vi "通信并与其他模块交互 (子VI).vi"() -> ()   [LabVIEW 2016, in "质控单元.lvlib"]
uses:
  <vilib>/Plasmionique/MB Master/MB_Master_TCP/MB_Master_TCP.lvclass
  D:/Program Files (x86)/National Instruments/LabVIEW 2016/vi.lib/Plasmionique/MB Master/MB_Master/MB_Master.lvclass
  <vilib>/Plasmionique/MB Master/MB_Master/MB_Master.lvclass
  <vilib>/Plasmionique/MB Master/MB Master.lvlib
  <vilib>/Utility/config.llb/NI_LVConfig.lvlib
panel:
  out "CODCr测量状态":u16[](array[numeric])
  out "CODMn测量状态":u16[](array[numeric])
  out "总氮测量状态":u16[](array[numeric])
  out "总磷测量状态":u16[](array[numeric])
  out "氨氮测量状态":u16[](array[numeric])
  out "通讯状态":bool
  out "待处理插入数量":i32
  out "元素":cluster{"命令":string}[](array[cluster])
  out "队列中元素数量":i32
  in  "starting address 6":u16
  in  "values 6":u16[](array[numeric])
  in  "starting address 5":u16
  in  "values 5":u16[](array[numeric])
  in  "starting address 4":u16
  in  "values 4":u16[](array[numeric])
  in  "starting address 3":u16
  in  "values 3":u16[](array[numeric])
  in  "starting address 2":u16
  in  "values 2":u16[](array[numeric])
  in  "values":u16[](array[numeric])
  in  "starting address":u16
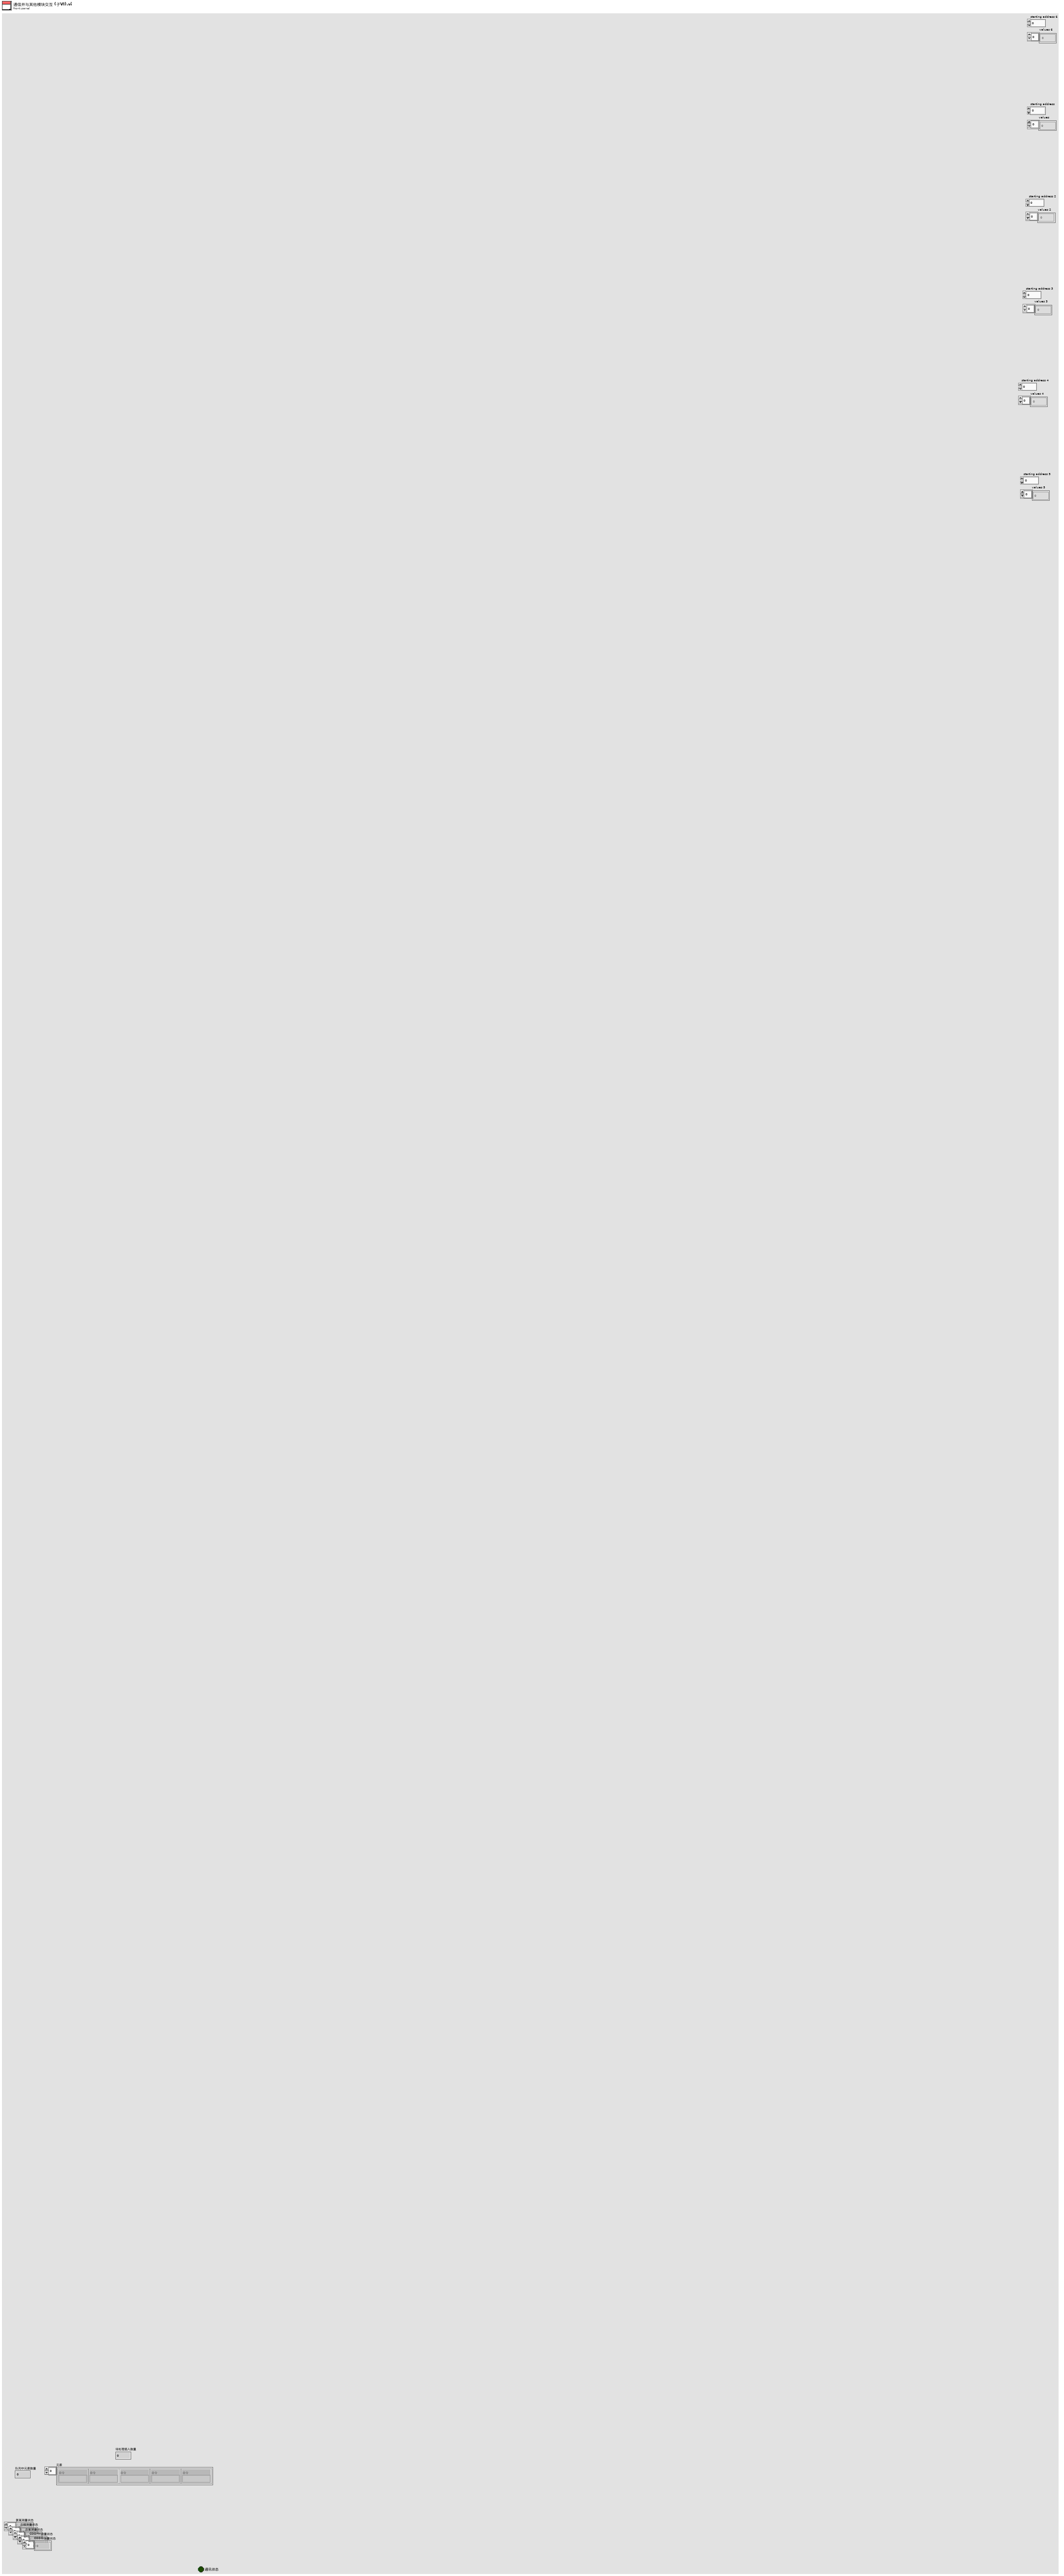
[diagram p1: front panel]
types:
  T1 = typedef "NI_LVConfig.lvlib/Config Data RefNum.ctl" = refnum<k1>
  T2 = cluster{"因子编码":u32, "单位":u16, "标样参考值":sgl, "水样数据时间":timestamp, "水样实测值":sgl, "水样数据标识":string, "标样数据时间":timestamp, "标样实测值":sgl, "标样数据标识":string, "空白数据时间":timestamp, "空白实测值":sgl, "空白数据标识":string, "零点核查数据时间":timestamp, "零点核查实测值":sgl, "零点核查数据标识":string, "跨度核查数据时间":timestamp, "跨度核查实测值":sgl, "跨度核查数据标识":string, "加标回收数据时间":timestamp, "加标回收实测值":sgl, "加标回收数据标识":string, "平行样数据时间":timestamp, "平行样实测值":sgl, "平行样数据标识":string}
  T3 = cluster{"系统时间":timestamp, "工作状态":enum16{"空闲", "水样测试", "标样核查", "零点核查", "跨度核查", "空白测试", "平行样测试", "加标回收", "空白校准", "标样校准", "初始化（清洗）"}, "测量模式":enum16{"待机", "连续模式", "周期模式", "定点模式", "受控模式", "手动模式"}, "告警代码":enum16{"无告警", "缺试剂告警", "缺水样告警", "缺蒸馏水告警", "缺标液告警", "仪表漏液告警", "标定异常告警", "超量程告警", "加热异常", "低试剂预警", "超上限告警", "超下限告警", "仪表内部其他异常", "滴定异常告警", "电极异常告警", "量程切换告警", "参数设置告警", "PH电极电位异常", "电导率电极异常", "浊度光度异常", "溶解氧电极异常", "溶解氧光强异常", "温度异常告警", "PH异常告警", "溶解氧异常告警", "电导率异常告警", "浊度异常告警", "叶绿素异常告警", "藻密度异常告警", "蓝绿藻异常告警", "ORP异常告警", "氨氮异常告警", "清洁刷异常告警", "SD卡异常告警", "蓝牙异常告警", "Wifi异常告警", "流程异常告警"}, "故障代码":enum16{"无故障", "电机故障", "温度故障", "通讯故障", "滴定故障"}, "日志代码":u16, "软件版本":u16, "F0":sgl, "F1":sgl, "F2":sgl, "F3":sgl, "T":sgl, "H":sgl, "id":u16, "flowid":u16, "量程":u16, "总磷控温温度1":sgl, "营养盐控温温度2":sgl, "ADC":sgl}
  T4 = cluster{"Registers[0]":u16, "Registers[1]":u16, "Registers[2]":u16, "Registers[3]":u16, "Registers[4]":u16, "Registers[5]":u16, "Registers[6]":u16, "Registers[7]":u16, "Registers[8]":u16, "Registers[9]":u16, "Registers[10]":u16, "Registers[11]":u16, "Registers[12]":u16, "Registers[13]":u16, "Registers[14]":u16, "Registers[15]":u16, "Registers[16]":u16, "Registers[17]":u16, "Registers[18]":u16, "Registers[19]":u16, "Registers[20]":u16, "Registers[21]":u16, "Registers[22]":u16, "Registers[23]":u16, "Registers[24]":u16, "Registers[25]":u16, "Registers[26]":u16, "Registers[27]":u16, "Registers[28]":u16, "Registers[29]":u16, "Registers[30]":u16, "Registers[31]":u16, "Registers[32]":u16, "Registers[33]":u16, "Registers[34]":u16, "Registers[35]":u16, "Registers[36]":u16, "Registers[37]":u16, "Registers[38]":u16, "Registers[39]":u16, "Registers[40]":u16, "Registers[41]":u16, "Registers[42]":u16, "Registers[43]":u16, "Registers[44]":u16, "Registers[45]":u16, "Registers[46]":u16, "Registers[47]":u16, "Registers[48]":u16, "Registers[49]":u16, "Registers[50]":u16, "Registers[51]":u16, "Registers[52]":u16, "Registers[53]":u16, "Registers[54]":u16, "Registers[55]":u16, "Registers[56]":u16}
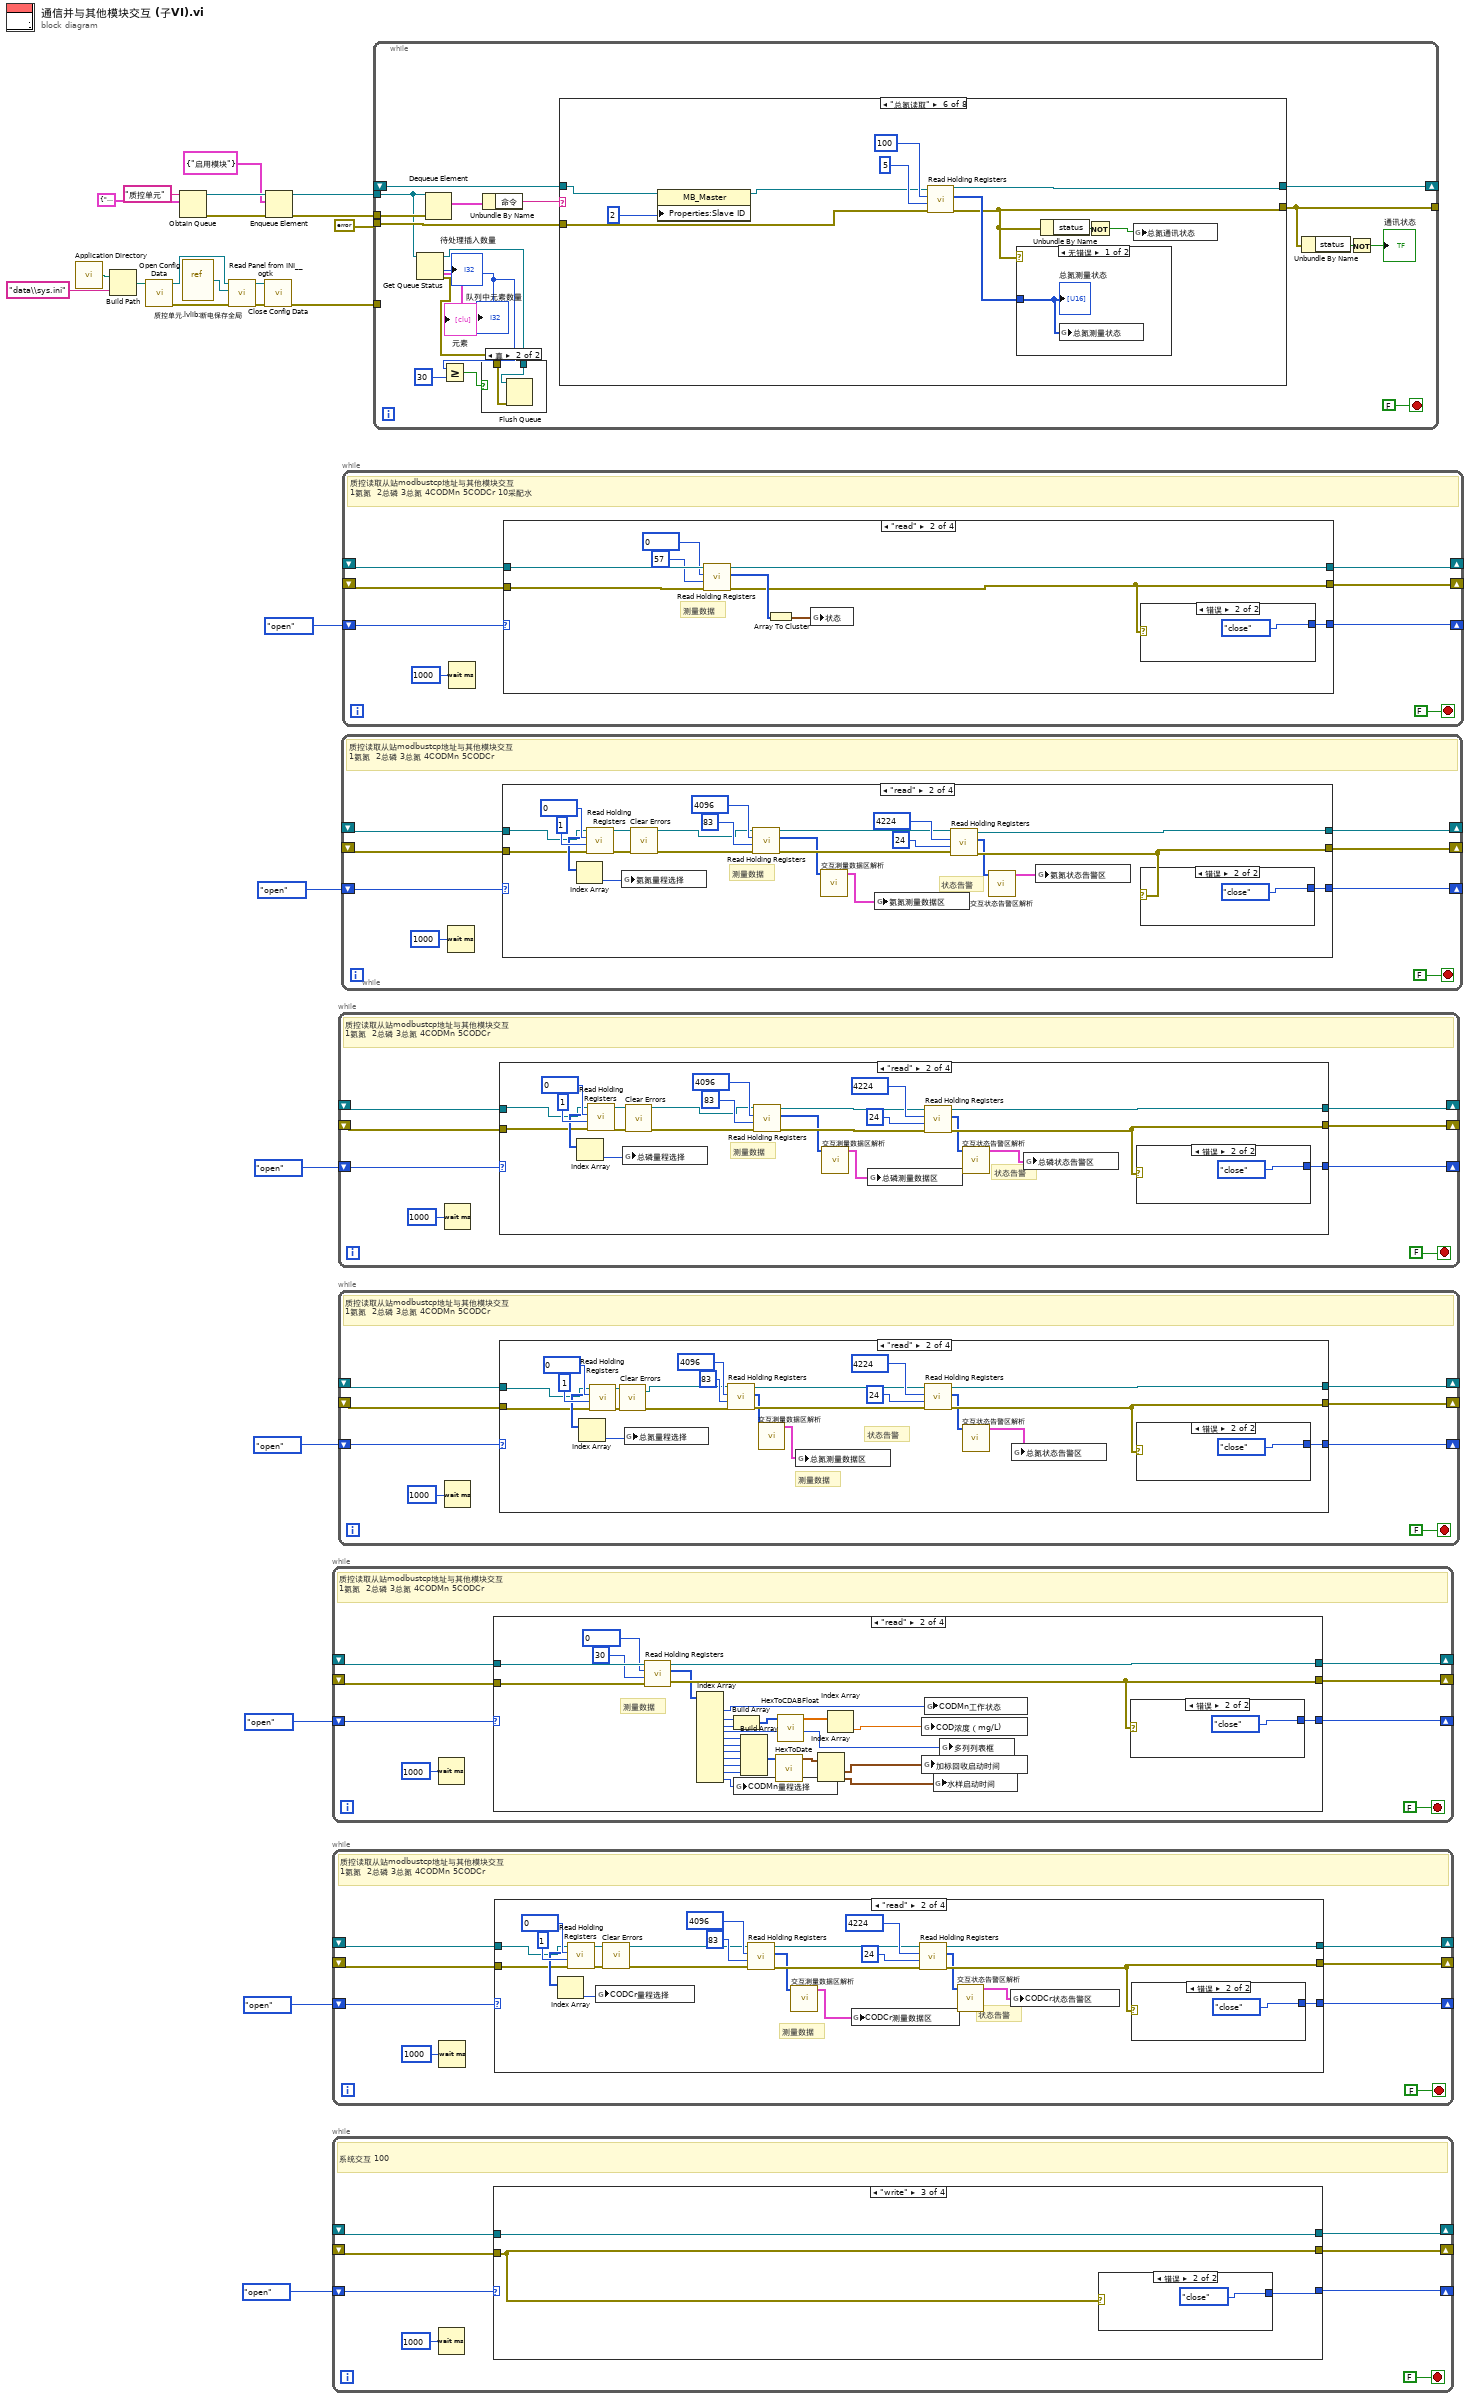
[diagram p0: block diagram]
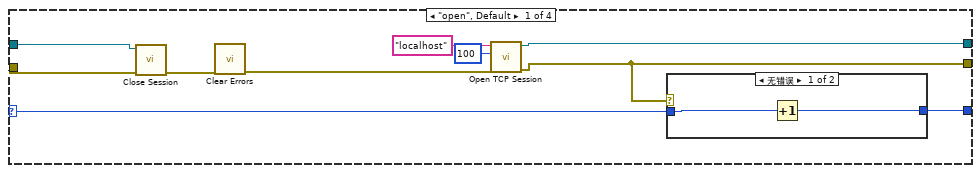
[diagram p2: hidden frame]
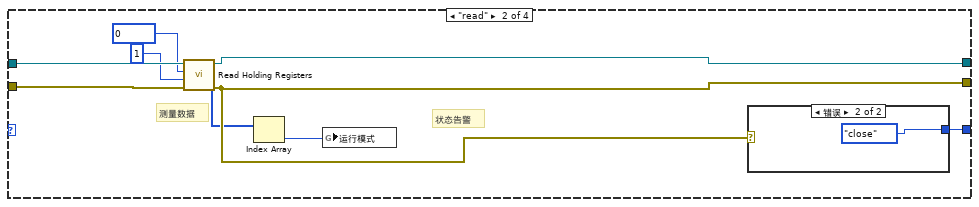
[diagram p4: hidden frame]
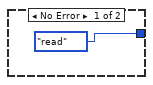
[diagram p5: hidden frame]
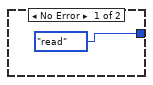
[diagram p6: hidden frame]
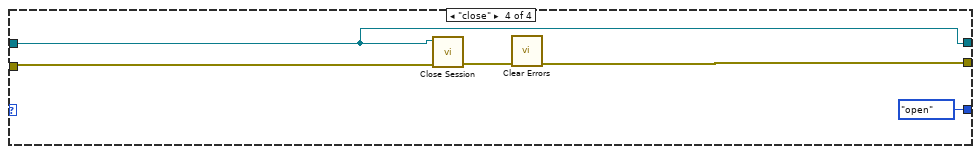
[diagram p7: hidden frame]
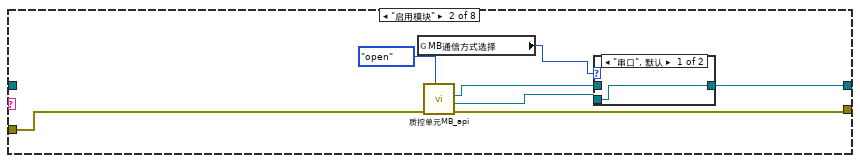
[diagram p10: hidden frame]
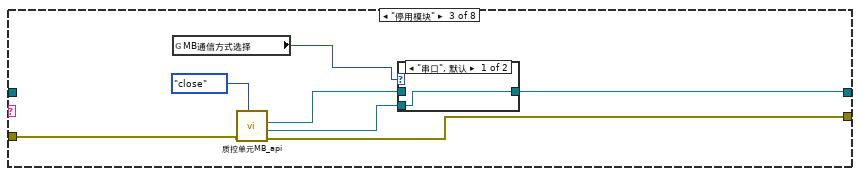
[diagram p12: hidden frame]
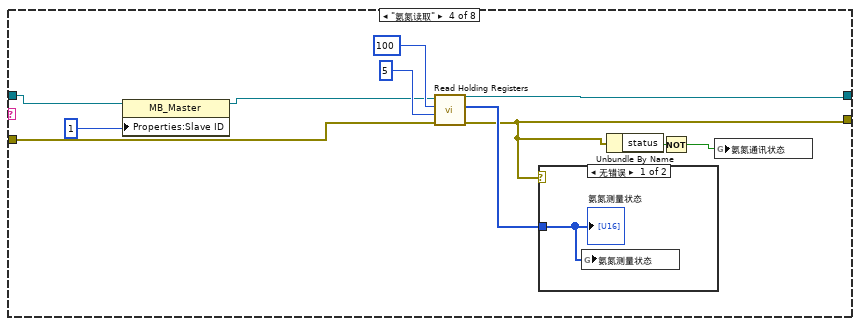
[diagram p14: hidden frame]
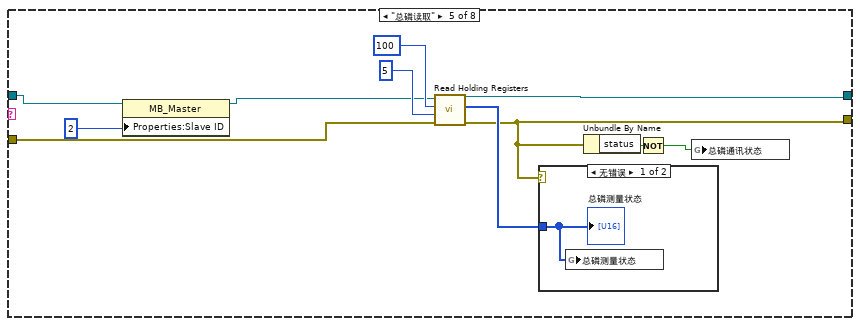
[diagram p16: hidden frame]
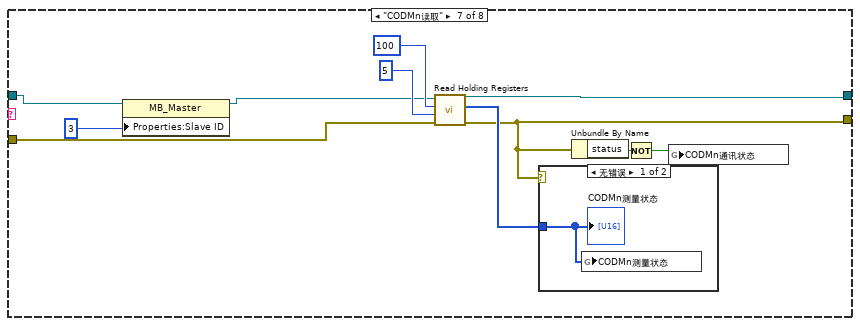
[diagram p19: hidden frame]
diagram:
  n1 = call <vilib>:"Application Directory.vi"() -> ("Application Directory"=w12:path)
  n2 = Build Path(base path=w12, name or relative path="data\\sys.ini" ("名称或相对路径")) -> (appended path=w10:path)
  n3 = call <vilib>:"Open Config Data.vi"("configuration file path"=w10) -> ("error out"=w6:errorcluster, "refnum"=w9:T1)  [unwired: 8 in, 1 out]
  n4 = Obtain Queue(name (unnamed)="质控单元" ("名称（未命名）"), element data type=cluster{"命令":string} {"命令"="启用模块"} ("元素")) -> (queue out=w15:refnum<queue>, error out=w14:errorcluster)  [unwired: 3 in, 1 out]
  n5 = vi-ref "质控单元.lvlib:断电保存全局.vi"() -> (w8:refnum<vi>)
  n6 = call <userlib>:"Read Panel from INI__ogtk.vi"("error in (no error)"=w6, "VI ref"=w8, "refnum"=w9) -> ("error out"=w5:errorcluster, "refnum out"=w7:T1)  [unwired: 7 in]
  n7 = call <vilib>:"Close Config Data.vi"("error in (no error)"=w5, "refnum"=w7) -> ("error out"=w1:errorcluster)  [unwired: 8 in, 1 out]
  n8 = Enqueue Element(queue=w15, element=cluster{"命令":string} {"命令"="启用模块"} ("元素"), error in (no error)=w14) -> (queue out=w4:refnum<queue>, error out=w3:errorcluster)  [unwired: 1 in, 1 out]
  n9 = while {
    shift-right: [w30] -> _
    shift-left: _ -> [w32]
    shift-right: [w29] -> _
    shift-left: _ -> [w31]
    shift-right: [w26] -> _
    shift-left: enum16{"open", "read", "write", "close"}."open" -> [w27]
    stop <- FALSE stop-if-true
    # "质控读取从站modbustcp地址与其他模块交互\n1氨氮  2总磷 3总氮 4CODMn 5CODCr"
    n10 = Wait (ms)(milliseconds to wait=u32 1000 ("等待时间（毫秒）")) -> ()  [unwired: 1 out]
    n11 = case shown="\"read\"" w27 {
      selector: w27 -> [w34 _ _ _]
      tunnel: w32 -> [w39 w71 w79 w87]
      tunnel: w31 -> [w38 w68 w78 w86]
      tunnel: [w40 w66 w77 w87] -> w30
      tunnel: [w35 w65 w76 w84] -> w29
      tunnel: [w33 w67 w80 enum16{"open", "read", "write", "close"}."open"] -> w26
      frame "open", Default {
        n12 = call-dynamic "Close Session.vi"("error in (no error)"=w38, "MB session in"=w39) -> ("error out"=w37:errorcluster)  [unwired: 9 in]
        n13 = call <vilib>:"Clear Errors.vi"("error in (no error)"=w37) -> ("error out"=w36:errorcluster)  [unwired: 5 in, 1 out]
        n14 = call <vilib>:"Open TCP Session.vi"("error in (no error)"=w36, "Port (502)"=u16 4, "IP Address"="localhost") -> ("error out"=w35:errorcluster, "MB_TCP session"=w40:refnum<class "MB_Master_TCP.lvclass">)  [unwired: 7 in]
        n15 = case shown="无错误" w35 {
          tunnel: w34 -> [w44 w45]
          tunnel: [w43 w45] -> w33
          frame No Error {
            n16 = Increment(x=w44) -> (x+1=w43:enum16{"open", "read", "write", "close"})
          }
          frame Error {
          }
        }
      }
      frame "read" {
        # "测量数据"
        n17 = call <vilib>:"Read Holding Registers.vi"("error in (no error)"=w68, "quantity"=u16 30, "starting address"=u16 0, "MB session in"=w71) -> ("error out"=w65:errorcluster, "Registers"=w64:u16[], "MB session out"=w66:refnum<class "MB_Master.lvclass">)  [unwired: 5 in]
        n18 = Index Array(array=w64) -> (element #1=w63:u16, element #2=w62:u16, element #3=w61:u16, element #4=w57:u16, element #5=w56:u16, element #6=w55:u16, element #7=w54:u16, element #8=w52:u16, element #9=w51:u16, element #10=w50:u16, element #11=w46:u16)  [unwired: 11 in]
        n19 = Build Array(w62, w61) -> (w60:u16[])
        n20 = global write "断电保存全局.vi" "CODMn量程选择"(w46) -> ()
        n21 = Build Array(w56, w55, w54, w52, w51, w50) -> (w53:u16[])
        n22 = call "HexToDate.vi"("数组"=w53) -> ("DATE"=w49:timestamp[])  [unwired: 10 in]
        n23 = call "HexToCDABFloat.vi"("数组"=w60) -> ("FLOAT"=w59:sgl[])  [unwired: 10 in]
        n24 = Index Array(array=w49) -> (element #1=w48:timestamp, element #2=w47:timestamp)  [unwired: 2 in]
        n25 = Index Array(array=w59) -> (element=w58:sgl)  [unwired: 1 in]
        n26 = global write "与CODMn交互全局.vi" "COD浓度（mg/L)"(w58) -> ()
        n27 = global write "与CODMn交互全局.vi" "加标回收启动时间"(w48) -> ()
        n28 = global write "与CODMn交互全局.vi" "CODMn工作状态"(w63) -> ()
        n29 = global write "与CODMn交互全局.vi" "水样启动时间"(w47) -> ()
        n30 = global write "与CODMn交互全局.vi" "多列列表框"(w57) -> ()
        n31 = case shown="错误" w65 {
          tunnel: [enum16{"open", "read", "write", "close"}."read" enum16{"open", "read", "write", "close"}."close"] -> w67
          frame No Error {
          }
          frame Error {
          }
        }
      }
      frame "write" {
        n32 = call <vilib>:"Write Multiple Registers.vi"("error in (no error)"=w78, "values"="values 4", "starting address"="starting address 4", "MB session in"=w79) -> ("error out"=w76:errorcluster, "MB session out"=w77:refnum<class "MB_Master.lvclass">)  [unwired: 6 in]
        n33 = case shown="错误" w76 {
          tunnel: [enum16{"open", "read", "write", "close"}."read" enum16{"open", "read", "write", "close"}."close"] -> w80
          frame No Error {
          }
          frame Error {
          }
        }
      }
      frame "close" {
        n34 = call-dynamic "Close Session.vi"("error in (no error)"=w86, "MB session in"=w87) -> ("error out"=w85:errorcluster)  [unwired: 9 in]
        n35 = call <vilib>:"Clear Errors.vi"("error in (no error)"=w85) -> ("error out"=w84:errorcluster)  [unwired: 5 in, 1 out]
      }
    }
  }
  n36 = while {
    shift-right: [w93] -> _
    shift-left: _ -> [w95]
    shift-right: [w92] -> _
    shift-left: _ -> [w94]
    shift-right: [w89] -> _
    shift-left: enum16{"open", "read", "write", "close"}."open" -> [w90]
    stop <- FALSE stop-if-true
    # "系统交互 100"
    n37 = Wait (ms)(milliseconds to wait=u32 1000 ("等待时间（毫秒）")) -> ()  [unwired: 1 out]
    n38 = case shown="\"write\"" w90 {
      selector: w90 -> [w97 _ _ _]
      tunnel: w95 -> [w102 w117 w121 w129]
      tunnel: w94 -> [w101 w114 w120 w128]
      tunnel: [w103 w112 w121 w129] -> w93
      tunnel: [w98 w111 w120 w126] -> w92
      tunnel: [w96 w113 w122 enum16{"open", "read", "write", "close"}."open"] -> w89
      frame "open", Default {
        n39 = call-dynamic "Close Session.vi"("error in (no error)"=w101, "MB session in"=w102) -> ("error out"=w100:errorcluster)  [unwired: 9 in]
        n40 = call <vilib>:"Clear Errors.vi"("error in (no error)"=w100) -> ("error out"=w99:errorcluster)  [unwired: 5 in, 1 out]
        n41 = call <vilib>:"Open TCP Session.vi"("error in (no error)"=w99, "Port (502)"=u16 100, "IP Address"="localhost") -> ("error out"=w98:errorcluster, "MB_TCP session"=w103:refnum<class "MB_Master_TCP.lvclass">)  [unwired: 7 in]
        n42 = case shown="无错误" w98 {
          tunnel: w97 -> [w107 w108]
          tunnel: [w106 w108] -> w96
          frame No Error {
            n43 = Increment(x=w107) -> (x+1=w106:enum16{"open", "read", "write", "close"})
          }
          frame Error {
          }
        }
      }
      frame "read" {
        # "状态告警"
        # "测量数据"
        n44 = call <vilib>:"Read Holding Registers.vi"("error in (no error)"=w114, "quantity"=u16 1, "starting address"=u16 0, "MB session in"=w117) -> ("error out"=w111:errorcluster, "Registers"=w110:u16[], "MB session out"=w112:refnum<class "MB_Master.lvclass">)  [unwired: 5 in]
        n45 = Index Array(array=w110) -> (element=w109:u16)  [unwired: 1 in]
        n46 = global write "系统交互.vi" "运行模式"(w109) -> ()
        n47 = case shown="错误" w111 {
          tunnel: [enum16{"open", "read", "write", "close"}."read" enum16{"open", "read", "write", "close"}."close"] -> w113
          frame No Error {
          }
          frame Error {
          }
        }
      }
      frame "write" {
        n48 = case shown="错误" w120 {
          tunnel: [enum16{"open", "read", "write", "close"}."read" enum16{"open", "read", "write", "close"}."close"] -> w122
          frame No Error {
          }
          frame Error {
          }
        }
      }
      frame "close" {
        n49 = call-dynamic "Close Session.vi"("error in (no error)"=w128, "MB session in"=w129) -> ("error out"=w127:errorcluster)  [unwired: 9 in]
        n50 = call <vilib>:"Clear Errors.vi"("error in (no error)"=w127) -> ("error out"=w126:errorcluster)  [unwired: 5 in, 1 out]
      }
    }
  }
  n51 = while {
    shift-right: [w135] -> _
    shift-left: _ -> [w137]
    shift-right: [w134] -> _
    shift-left: _ -> [w136]
    shift-right: [w131] -> _
    shift-left: enum16{"open", "read", "write", "close"}."open" -> [w132]
    stop <- FALSE stop-if-true
    # "质控读取从站modbustcp地址与其他模块交互\n1氨氮  2总磷 3总氮 4CODMn 5CODCr"
    n52 = Wait (ms)(milliseconds to wait=u32 1000 ("等待时间（毫秒）")) -> ()  [unwired: 1 out]
    n53 = case shown="\"read\"" w132 {
      selector: w132 -> [w139 _ _ _]
      tunnel: w137 -> [w144 w155 w180 w188]
      tunnel: w136 -> [w143 w154 w179 w187]
      tunnel: [w145 w165 w178 w188] -> w135
      tunnel: [w140 w164 w177 w185] -> w134
      tunnel: [w138 w170 w181 enum16{"open", "read", "write", "close"}."open"] -> w131
      frame "open", Default {
        n54 = call-dynamic "Close Session.vi"("error in (no error)"=w143, "MB session in"=w144) -> ("error out"=w142:errorcluster)  [unwired: 9 in]
        n55 = call <vilib>:"Clear Errors.vi"("error in (no error)"=w142) -> ("error out"=w141:errorcluster)  [unwired: 5 in, 1 out]
        n56 = call <vilib>:"Open TCP Session.vi"("error in (no error)"=w141, "Port (502)"=u16 5, "IP Address"="localhost") -> ("error out"=w140:errorcluster, "MB_TCP session"=w145:refnum<class "MB_Master_TCP.lvclass">)  [unwired: 7 in]
        n57 = case shown="无错误" w140 {
          tunnel: w139 -> [w149 w150]
          tunnel: [w148 w150] -> w138
          frame No Error {
            n58 = Increment(x=w149) -> (x+1=w148:enum16{"open", "read", "write", "close"})
          }
          frame Error {
          }
        }
      }
      frame "read" {
        # "状态告警"
        # "测量数据"
        n59 = call <vilib>:"Read Holding Registers.vi"("error in (no error)"=w154, "quantity"=u16 1, "starting address"=u16 0, "MB session in"=w155) -> ("error out"=w153:errorcluster, "Registers"=w157:u16[], "MB session out"=w152:refnum<class "MB_Master.lvclass">)  [unwired: 5 in]
        n60 = Index Array(array=w157) -> (element=w156:u16)  [unwired: 1 in]
        n61 = global write "断电保存全局.vi" "CODCr量程选择"(w156) -> ()
        n62 = call <vilib>:"Clear Errors.vi"("error in (no error)"=w153) -> ("error out"=w151:errorcluster)  [unwired: 5 in, 1 out]
        n63 = call <vilib>:"Read Holding Registers.vi"("error in (no error)"=w151, "quantity"=u16 83, "starting address"=u16 4096, "MB session in"=w152) -> ("error out"=w166:errorcluster, "Registers"=w163:u16[], "MB session out"=w167:refnum<class "MB_Master.lvclass">)  [unwired: 5 in]
        n64 = call "交互测量数据区解析.vi"("数组"=w163) -> ("测量数据区"=w161:T2)  [unwired: 10 in]
        n65 = global write "与CODCr交互全局.vi" "CODCr测量数据区"(w161) -> ()
        n66 = call <vilib>:"Read Holding Registers.vi"("error in (no error)"=w166, "quantity"=u16 24, "starting address"=u16 4224, "MB session in"=w167) -> ("error out"=w164:errorcluster, "Registers"=w162:u16[], "MB session out"=w165:refnum<class "MB_Master.lvclass">)  [unwired: 5 in]
        n67 = call "交互状态告警区解析.vi"("数组"=w162) -> ("状态告警区"=w160:T3)  [unwired: 10 in]
        n68 = global write "与CODCr交互全局.vi" "CODCr状态告警区"(w160) -> ()
        n69 = case shown="错误" w164 {
          tunnel: [enum16{"open", "read", "write", "close"}."read" enum16{"open", "read", "write", "close"}."close"] -> w170
          frame No Error {
          }
          frame Error {
          }
        }
      }
      frame "write" {
        n70 = call <vilib>:"Write Multiple Registers.vi"("error in (no error)"=w179, "values"="values 5", "starting address"="starting address 5", "MB session in"=w180) -> ("error out"=w177:errorcluster, "MB session out"=w178:refnum<class "MB_Master.lvclass">)  [unwired: 6 in]
        n71 = case shown="错误" w177 {
          tunnel: [enum16{"open", "read", "write", "close"}."read" enum16{"open", "read", "write", "close"}."close"] -> w181
          frame No Error {
          }
          frame Error {
          }
        }
      }
      frame "close" {
        n72 = call-dynamic "Close Session.vi"("error in (no error)"=w187, "MB session in"=w188) -> ("error out"=w186:errorcluster)  [unwired: 9 in]
        n73 = call <vilib>:"Clear Errors.vi"("error in (no error)"=w186) -> ("error out"=w185:errorcluster)  [unwired: 5 in, 1 out]
      }
    }
  }
  n74 = while {
    shift-right: [w194] -> _
    shift-left: _ -> [w196]
    shift-right: [w193] -> _
    shift-left: _ -> [w195]
    shift-right: [w190] -> _
    shift-left: enum16{"open", "read", "write", "close"}."open" -> [w191]
    stop <- FALSE stop-if-true
    # "质控读取从站modbustcp地址与其他模块交互\n1氨氮  2总磷 3总氮 4CODMn 5CODCr"
    n75 = Wait (ms)(milliseconds to wait=u32 1000 ("等待时间（毫秒）")) -> ()  [unwired: 1 out]
    n76 = case shown="\"read\"" w191 {
      selector: w191 -> [w198 _ _ _]
      tunnel: w196 -> [w203 w214 w239 w247]
      tunnel: w195 -> [w202 w213 w238 w246]
      tunnel: [w204 w224 w237 w247] -> w194
      tunnel: [w199 w223 w236 w244] -> w193
      tunnel: [w197 w229 w240 enum16{"open", "read", "write", "close"}."open"] -> w190
      frame "open", Default {
        n77 = call-dynamic "Close Session.vi"("error in (no error)"=w202, "MB session in"=w203) -> ("error out"=w201:errorcluster)  [unwired: 9 in]
        n78 = call <vilib>:"Clear Errors.vi"("error in (no error)"=w201) -> ("error out"=w200:errorcluster)  [unwired: 5 in, 1 out]
        n79 = call <vilib>:"Open TCP Session.vi"("error in (no error)"=w200, "Port (502)"=u16 2, "IP Address"="localhost") -> ("error out"=w199:errorcluster, "MB_TCP session"=w204:refnum<class "MB_Master_TCP.lvclass">)  [unwired: 7 in]
        n80 = case shown="无错误" w199 {
          tunnel: w198 -> [w208 w209]
          tunnel: [w207 w209] -> w197
          frame No Error {
            n81 = Increment(x=w208) -> (x+1=w207:enum16{"open", "read", "write", "close"})
          }
          frame Error {
          }
        }
      }
      frame "read" {
        # "状态告警"
        # "测量数据"
        n82 = call <vilib>:"Read Holding Registers.vi"("error in (no error)"=w213, "quantity"=u16 1, "starting address"=u16 0, "MB session in"=w214) -> ("error out"=w211:errorcluster, "Registers"=w216:u16[], "MB session out"=w212:refnum<class "MB_Master.lvclass">)  [unwired: 5 in]
        n83 = Index Array(array=w216) -> (element=w215:u16)  [unwired: 1 in]
        n84 = global write "断电保存全局.vi" "总磷量程选择"(w215) -> ()
        n85 = call <vilib>:"Clear Errors.vi"("error in (no error)"=w211) -> ("error out"=w210:errorcluster)  [unwired: 5 in, 1 out]
        n86 = call <vilib>:"Read Holding Registers.vi"("error in (no error)"=w210, "quantity"=u16 83, "starting address"=u16 4096, "MB session in"=w212) -> ("error out"=w225:errorcluster, "Registers"=w222:u16[], "MB session out"=w226:refnum<class "MB_Master.lvclass">)  [unwired: 5 in]
        n87 = call "交互测量数据区解析.vi"("数组"=w222) -> ("测量数据区"=w220:T2)  [unwired: 10 in]
        n88 = global write "与总磷交互全局.vi" "总磷测量数据区"(w220) -> ()
        n89 = call <vilib>:"Read Holding Registers.vi"("error in (no error)"=w225, "quantity"=u16 24, "starting address"=u16 4224, "MB session in"=w226) -> ("error out"=w223:errorcluster, "Registers"=w221:u16[], "MB session out"=w224:refnum<class "MB_Master.lvclass">)  [unwired: 5 in]
        n90 = call "交互状态告警区解析.vi"("数组"=w221) -> ("状态告警区"=w219:T3)  [unwired: 10 in]
        n91 = global write "与总磷交互全局.vi" "总磷状态告警区"(w219) -> ()
        n92 = case shown="错误" w223 {
          tunnel: [enum16{"open", "read", "write", "close"}."read" enum16{"open", "read", "write", "close"}."close"] -> w229
          frame No Error {
          }
          frame Error {
          }
        }
      }
      frame "write" {
        n93 = call <vilib>:"Write Multiple Registers.vi"("error in (no error)"=w238, "values"="values 2", "starting address"="starting address 2", "MB session in"=w239) -> ("error out"=w236:errorcluster, "MB session out"=w237:refnum<class "MB_Master.lvclass">)  [unwired: 6 in]
        n94 = case shown="错误" w236 {
          tunnel: [enum16{"open", "read", "write", "close"}."read" enum16{"open", "read", "write", "close"}."close"] -> w240
          frame No Error {
          }
          frame Error {
          }
        }
      }
      frame "close" {
        n95 = call-dynamic "Close Session.vi"("error in (no error)"=w246, "MB session in"=w247) -> ("error out"=w245:errorcluster)  [unwired: 9 in]
        n96 = call <vilib>:"Clear Errors.vi"("error in (no error)"=w245) -> ("error out"=w244:errorcluster)  [unwired: 5 in, 1 out]
      }
    }
  }
  n97 = while {
    shift-right: [w253] -> _
    shift-left: _ -> [w255]
    shift-right: [w252] -> _
    shift-left: _ -> [w254]
    shift-right: [w249] -> _
    shift-left: enum16{"open", "read", "write", "close"}."open" -> [w250]
    stop <- FALSE stop-if-true
    # "质控读取从站modbustcp地址与其他模块交互\n1氨氮  2总磷 3总氮 4CODMn 5CODCr"
    n98 = Wait (ms)(milliseconds to wait=u32 1000 ("等待时间（毫秒）")) -> ()  [unwired: 1 out]
    n99 = case shown="\"read\"" w250 {
      selector: w250 -> [w257 _ _ _]
      tunnel: w255 -> [w262 w273 w298 w306]
      tunnel: w254 -> [w261 w272 w297 w305]
      tunnel: [w263 w283 w296 w306] -> w253
      tunnel: [w258 w282 w295 w303] -> w252
      tunnel: [w256 w288 w299 enum16{"open", "read", "write", "close"}."open"] -> w249
      frame "open", Default {
        n100 = call-dynamic "Close Session.vi"("error in (no error)"=w261, "MB session in"=w262) -> ("error out"=w260:errorcluster)  [unwired: 9 in]
        n101 = call <vilib>:"Clear Errors.vi"("error in (no error)"=w260) -> ("error out"=w259:errorcluster)  [unwired: 5 in, 1 out]
        n102 = call <vilib>:"Open TCP Session.vi"("error in (no error)"=w259, "Port (502)"=u16 3, "IP Address"="localhost") -> ("error out"=w258:errorcluster, "MB_TCP session"=w263:refnum<class "MB_Master_TCP.lvclass">)  [unwired: 7 in]
        n103 = case shown="无错误" w258 {
          tunnel: w257 -> [w267 w268]
          tunnel: [w266 w268] -> w256
          frame No Error {
            n104 = Increment(x=w267) -> (x+1=w266:enum16{"open", "read", "write", "close"})
          }
          frame Error {
          }
        }
      }
      frame "read" {
        # "状态告警"
        # "测量数据"
        n105 = call <vilib>:"Read Holding Registers.vi"("error in (no error)"=w272, "quantity"=u16 1, "starting address"=u16 0, "MB session in"=w273) -> ("error out"=w270:errorcluster, "Registers"=w275:u16[], "MB session out"=w271:refnum<class "MB_Master.lvclass">)  [unwired: 5 in]
        n106 = Index Array(array=w275) -> (element=w274:u16)  [unwired: 1 in]
        n107 = call <vilib>:"Clear Errors.vi"("error in (no error)"=w270) -> ("error out"=w269:errorcluster)  [unwired: 5 in, 1 out]
        n108 = global write "断电保存全局.vi" "总氮量程选择"(w274) -> ()
        n109 = call <vilib>:"Read Holding Registers.vi"("error in (no error)"=w269, "quantity"=u16 83, "starting address"=u16 4096, "MB session in"=w271) -> ("error out"=w284:errorcluster, "Registers"=w281:u16[], "MB session out"=w285:refnum<class "MB_Master.lvclass">)  [unwired: 5 in]
        n110 = call "交互测量数据区解析.vi"("数组"=w281) -> ("测量数据区"=w279:T2)  [unwired: 10 in]
        n111 = global write "与总氮交互全局.vi" "总氮测量数据区"(w279) -> ()
        n112 = call <vilib>:"Read Holding Registers.vi"("error in (no error)"=w284, "quantity"=u16 24, "starting address"=u16 4224, "MB session in"=w285) -> ("error out"=w282:errorcluster, "Registers"=w280:u16[], "MB session out"=w283:refnum<class "MB_Master.lvclass">)  [unwired: 5 in]
        n113 = call "交互状态告警区解析.vi"("数组"=w280) -> ("状态告警区"=w278:T3)  [unwired: 10 in]
        n114 = global write "与总氮交互全局.vi" "总氮状态告警区"(w278) -> ()
        n115 = case shown="错误" w282 {
          tunnel: [enum16{"open", "read", "write", "close"}."read" enum16{"open", "read", "write", "close"}."close"] -> w288
          frame No Error {
          }
          frame Error {
          }
        }
      }
      frame "write" {
        n116 = call <vilib>:"Write Multiple Registers.vi"("error in (no error)"=w297, "values"="values 3", "starting address"="starting address 3", "MB session in"=w298) -> ("error out"=w295:errorcluster, "MB session out"=w296:refnum<class "MB_Master.lvclass">)  [unwired: 6 in]
        n117 = case shown="错误" w295 {
          tunnel: [enum16{"open", "read", "write", "close"}."read" enum16{"open", "read", "write", "close"}."close"] -> w299
          frame No Error {
          }
          frame Error {
          }
        }
      }
      frame "close" {
        n118 = call-dynamic "Close Session.vi"("error in (no error)"=w305, "MB session in"=w306) -> ("error out"=w304:errorcluster)  [unwired: 9 in]
        n119 = call <vilib>:"Clear Errors.vi"("error in (no error)"=w304) -> ("error out"=w303:errorcluster)  [unwired: 5 in, 1 out]
      }
    }
  }
  n120 = while {
    shift-right: [w312] -> _
    shift-left: _ -> [w314]
    shift-right: [w311] -> _
    shift-left: _ -> [w313]
    shift-right: [w308] -> _
    shift-left: enum16{"open", "read", "write", "close"}."open" -> [w309]
    stop <- FALSE stop-if-true
    # "质控读取从站modbustcp地址与其他模块交互\n1氨氮  2总磷 3总氮 4CODMn 5CODCr"
    n121 = Wait (ms)(milliseconds to wait=u32 1000 ("等待时间（毫秒）")) -> ()  [unwired: 1 out]
    n122 = case shown="\"read\"" w309 {
      selector: w309 -> [w316 _ _ _]
      tunnel: w314 -> [w321 w332 w357 w365]
      tunnel: w313 -> [w320 w331 w356 w364]
      tunnel: [w322 w342 w355 w365] -> w312
      tunnel: [w317 w341 w354 w362] -> w311
      tunnel: [w315 w347 w358 enum16{"open", "read", "write", "close"}."open"] -> w308
      frame "open", Default {
        n123 = call-dynamic "Close Session.vi"("error in (no error)"=w320, "MB session in"=w321) -> ("error out"=w319:errorcluster)  [unwired: 9 in]
        n124 = call <vilib>:"Clear Errors.vi"("error in (no error)"=w319) -> ("error out"=w318:errorcluster)  [unwired: 5 in, 1 out]
        n125 = call <vilib>:"Open TCP Session.vi"("error in (no error)"=w318, "Port (502)"=u16 1, "IP Address"="localhost") -> ("error out"=w317:errorcluster, "MB_TCP session"=w322:refnum<class "MB_Master_TCP.lvclass">)  [unwired: 7 in]
        n126 = case shown="无错误" w317 {
          tunnel: w316 -> [w326 w327]
          tunnel: [w325 w327] -> w315
          frame No Error {
            n127 = Increment(x=w326) -> (x+1=w325:enum16{"open", "read", "write", "close"})
          }
          frame Error {
          }
        }
      }
      frame "read" {
        # "状态告警"
        # "测量数据"
        n128 = call <vilib>:"Read Holding Registers.vi"("error in (no error)"=w331, "quantity"=u16 1, "starting address"=u16 0, "MB session in"=w332) -> ("error out"=w329:errorcluster, "Registers"=w334:u16[], "MB session out"=w330:refnum<class "MB_Master.lvclass">)  [unwired: 5 in]
        n129 = Index Array(array=w334) -> (element=w333:u16)  [unwired: 1 in]
        n130 = global write "断电保存全局.vi" "氨氮量程选择"(w333) -> ()
        n131 = call <vilib>:"Clear Errors.vi"("error in (no error)"=w329) -> ("error out"=w328:errorcluster)  [unwired: 5 in, 1 out]
        n132 = call <vilib>:"Read Holding Registers.vi"("error in (no error)"=w328, "quantity"=u16 83, "starting address"=u16 4096, "MB session in"=w330) -> ("error out"=w343:errorcluster, "Registers"=w340:u16[], "MB session out"=w344:refnum<class "MB_Master.lvclass">)  [unwired: 5 in]
        n133 = call "交互测量数据区解析.vi"("数组"=w340) -> ("测量数据区"=w339:T2)  [unwired: 10 in]
        n134 = global write "与氨氮交互全局.vi" "氨氮测量数据区"(w339) -> ()
        n135 = call <vilib>:"Read Holding Registers.vi"("error in (no error)"=w343, "quantity"=u16 24, "starting address"=u16 4224, "MB session in"=w344) -> ("error out"=w341:errorcluster, "Registers"=w338:u16[], "MB session out"=w342:refnum<class "MB_Master.lvclass">)  [unwired: 5 in]
        n136 = call "交互状态告警区解析.vi"("数组"=w338) -> ("状态告警区"=w337:T3)  [unwired: 10 in]
        n137 = global write "与氨氮交互全局.vi" "氨氮状态告警区"(w337) -> ()
        n138 = case shown="错误" w341 {
          tunnel: [enum16{"open", "read", "write", "close"}."read" enum16{"open", "read", "write", "close"}."close"] -> w347
          frame No Error {
          }
          frame Error {
          }
        }
      }
      frame "write" {
        n139 = call <vilib>:"Write Multiple Registers.vi"("error in (no error)"=w356, "values"="values", "starting address"="starting address", "MB session in"=w357) -> ("error out"=w354:errorcluster, "MB session out"=w355:refnum<class "MB_Master.lvclass">)  [unwired: 6 in]
        n140 = case shown="错误" w354 {
          tunnel: [enum16{"open", "read", "write", "close"}."read" enum16{"open", "read", "write", "close"}."close"] -> w358
          frame No Error {
          }
          frame Error {
          }
        }
      }
      frame "close" {
        n141 = call-dynamic "Close Session.vi"("error in (no error)"=w364, "MB session in"=w365) -> ("error out"=w363:errorcluster)  [unwired: 9 in]
        n142 = call <vilib>:"Clear Errors.vi"("error in (no error)"=w363) -> ("error out"=w362:errorcluster)  [unwired: 5 in, 1 out]
      }
    }
  }
  n143 = while {
    shift-right: [w371] -> _
    shift-left: _ -> [w373]
    shift-right: [w370] -> _
    shift-left: _ -> [w372]
    shift-right: [w367] -> _
    shift-left: enum16{"open", "read", "write", "close"}."open" -> [w368]
    stop <- FALSE stop-if-true
    # "质控读取从站modbustcp地址与其他模块交互\n1氨氮  2总磷 3总氮 4CODMn 5CODCr 10采配水"
    n144 = Wait (ms)(milliseconds to wait=u32 1000 ("等待时间（毫秒）")) -> ()  [unwired: 1 out]
    n145 = case shown="\"read\"" w368 {
      selector: w368 -> [w375 _ _ _]
      tunnel: w373 -> [w380 w395 w403 w411]
      tunnel: w372 -> [w379 w392 w402 w410]
      tunnel: [w381 w388 w401 w411] -> w371
      tunnel: [w376 w387 w400 w408] -> w370
      tunnel: [w374 w391 w404 enum16{"open", "read", "write", "close"}."open"] -> w367
      frame "open", Default {
        n146 = call-dynamic "Close Session.vi"("error in (no error)"=w379, "MB session in"=w380) -> ("error out"=w378:errorcluster)  [unwired: 9 in]
        n147 = call <vilib>:"Clear Errors.vi"("error in (no error)"=w378) -> ("error out"=w377:errorcluster)  [unwired: 5 in, 1 out]
        n148 = call <vilib>:"Open TCP Session.vi"("error in (no error)"=w377, "Port (502)"=u16 10, "IP Address"="localhost") -> ("error out"=w376:errorcluster, "MB_TCP session"=w381:refnum<class "MB_Master_TCP.lvclass">)  [unwired: 7 in]
        n149 = case shown="无错误" w376 {
          tunnel: w375 -> [w385 w386]
          tunnel: [w384 w386] -> w374
          frame No Error {
            n150 = Increment(x=w385) -> (x+1=w384:enum16{"open", "read", "write", "close"})
          }
          frame Error {
          }
        }
      }
      frame "read" {
        # "测量数据"
        n151 = call <vilib>:"Read Holding Registers.vi"("error in (no error)"=w392, "quantity"=u16 57, "starting address"=u16 0, "MB session in"=w395) -> ("error out"=w387:errorcluster, "Registers"=w390:u16[], "MB session out"=w388:refnum<class "MB_Master.lvclass">)  [unwired: 5 in]
        n152 = Array To Cluster(array=w390) -> (cluster=w389:T4)
        n153 = global write "与采配水交互全局.vi" "状态"(w389) -> ()
        n154 = case shown="错误" w387 {
          tunnel: [enum16{"open", "read", "write", "close"}."read" enum16{"open", "read", "write", "close"}."close"] -> w391
          frame No Error {
          }
          frame Error {
          }
        }
      }
      frame "write" {
        n155 = call <vilib>:"Write Multiple Registers.vi"("error in (no error)"=w402, "values"="values 6", "starting address"="starting address 6", "MB session in"=w403) -> ("error out"=w400:errorcluster, "MB session out"=w401:refnum<class "MB_Master.lvclass">)  [unwired: 6 in]
        n156 = case shown="错误" w400 {
          tunnel: [enum16{"open", "read", "write", "close"}."read" enum16{"open", "read", "write", "close"}."close"] -> w404
          frame No Error {
          }
          frame Error {
          }
        }
      }
      frame "close" {
        n157 = call-dynamic "Close Session.vi"("error in (no error)"=w410, "MB session in"=w411) -> ("error out"=w409:errorcluster)  [unwired: 9 in]
        n158 = call <vilib>:"Clear Errors.vi"("error in (no error)"=w409) -> ("error out"=w408:errorcluster)  [unwired: 5 in, 1 out]
      }
    }
  }
  n159 = while {
    tunnel: w4 -> [w419]
    tunnel: w3 -> [w428]
    tunnel: [w420] -> _
    shift-right: [w424] -> _
    shift-left: _ -> [w423]
    tunnel: errorcluster {"status"=FALSE, "code"=0, "source"=""} ("error out") -> [w422]
    tunnel: w1 -> [_]
    stop <- FALSE stop-if-true
    n160 = Get Queue Status(queue=w419) -> (queue out=w413:refnum<queue>, # pending insert=→"待处理插入数量":i32, error out=w412:errorcluster, # elements in queue=w416:i32, elements=→"元素":cluster{"命令":string}[])  [unwired: 2 in, 3 out]
    "队列中元素数量" <- w416
    n161 = Dequeue Element(queue=w419, error in (no error)=w428) -> (element=w427:cluster{"命令":string})  [unwired: 1 in, 3 out]
    n162 = Greater Or Equal?(x=w416, y=30) -> (x >= y?=w414:bool)
    n163 = case shown="真" w414 {
      tunnel: w413 -> [_ w431]
      tunnel: w412 -> [_ w430]
      frame False {
      }
      frame True {
        n164 = Flush Queue(queue=w431, error in (no error)=w430) -> ()  [unwired: 3 out]
      }
    }
    n165 = Unbundle By Name(w427) -> ("命令"=w426:string)
    n166 = case shown="\"总氮读取\"" w426 {
      tunnel: [w433 w435 w445 w458 w470 w482 w494 w506] -> w424
      tunnel: [w432 w440 w447 w453 w464 w476 w488 w500] -> w420
      tunnel: w423 -> [w433 _ _ w456 w468 w480 w492 w504]
      tunnel: w422 -> [w432 w438 w448 w462 w474 w486 w498 w510]
      frame Default {
      }
      frame "启用模块" {
        n167 = global read "断电保存全局.vi" "MB通信方式选择"() -> (w434:enum16{"串口", "TCP"})
        n168 = call "质控单元MB_api.vi"("STEP"=enum16{"open", "read", "write", "close"}."open", "Error in"=w438) -> ("error out"=w440:errorcluster, "MB session out"=w436:refnum<class "MB_Master.lvclass">, "MB_TCP session"=w437:refnum<class "MB_Master_TCP.lvclass">)  [unwired: 6 in, 1 out]
        n169 = case shown="\"串口\", 默认" w434 {
          tunnel: w437 -> [_ w442]
          tunnel: w436 -> [w441 _]
          tunnel: [w441 w442] -> w435
          frame "串口", Default {
          }
          frame "TCP" {
          }
        }
      }
      frame "停用模块" {
        n170 = global read "断电保存全局.vi" "MB通信方式选择"() -> (w443:enum16{"串口", "TCP"})
        n171 = call "质控单元MB_api.vi"("STEP"=enum16{"open", "read", "write", "close"}."close", "Error in"=w448) -> ("error out"=w447:errorcluster, "MB session out"=w446:refnum<class "MB_Master.lvclass">, "MB_TCP session"=w444:refnum<class "MB_Master_TCP.lvclass">)  [unwired: 6 in, 1 out]
        n172 = case shown="\"串口\", 默认" w443 {
          tunnel: w444 -> [_ w451]
          tunnel: w446 -> [w450 _]
          tunnel: [w450 w451] -> w445
          frame "串口", Default {
          }
          frame "TCP" {
          }
        }
      }
      frame "氨氮读取" {
        n173 = property class="MB_Master"(reference=w456, "Properties:Slave ID"=u8 1 ("Slave ID")) -> (reference out=w455:refnum<class "MB_Master.lvclass">)  [unwired: 1 in, 1 out]
        n174 = call <vilib>:"Read Holding Registers.vi"("error in (no error)"=w462, "quantity"=u16 5 ("number of holding registers"), "starting address"=u16 100, "MB session in"=w455) -> ("error out"=w453:errorcluster, "Registers"=w459:u16[], "MB session out"=w458:refnum<class "MB_Master.lvclass">)  [unwired: 5 in]
        n175 = case shown="无错误" w453 {
          tunnel: w459 -> [w463 _]
          frame No Error {
            n176 = global write "质控内部交互全局.vi" "氨氮测量状态"(w463) -> ()
            "氨氮测量状态" <- w463
          }
          frame Error {
          }
        }
        n177 = Unbundle By Name(w453) -> ("status"=w454:bool)
        n178 = Not(x=w454) -> (.not. x?=w452:bool)
        n179 = global write "质控内部交互全局.vi" "氨氮通讯状态"(w452) -> ()
      }
      frame "总磷读取" {
        n180 = property class="MB_Master"(reference=w468, "Properties:Slave ID"=u8 2 ("Slave ID")) -> (reference out=w467:refnum<class "MB_Master.lvclass">)  [unwired: 1 in, 1 out]
        n181 = call <vilib>:"Read Holding Registers.vi"("error in (no error)"=w474, "quantity"=u16 5 ("number of holding registers"), "starting address"=u16 100, "MB session in"=w467) -> ("error out"=w464:errorcluster, "Registers"=w471:u16[], "MB session out"=w470:refnum<class "MB_Master.lvclass">)  [unwired: 5 in]
        n182 = case shown="无错误" w464 {
          tunnel: w471 -> [w475 _]
          frame No Error {
            n183 = global write "质控内部交互全局.vi" "总磷测量状态"(w475) -> ()
            "总磷测量状态" <- w475
          }
          frame Error {
          }
        }
        n184 = Unbundle By Name(w464) -> ("status"=w466:bool)
        n185 = Not(x=w466) -> (.not. x?=w465:bool)
        n186 = global write "质控内部交互全局.vi" "总磷通讯状态"(w465) -> ()
      }
      frame "总氮读取" {
        n187 = property class="MB_Master"(reference=w480, "Properties:Slave ID"=u8 2 ("Slave ID")) -> (reference out=w479:refnum<class "MB_Master.lvclass">)  [unwired: 1 in, 1 out]
        n188 = call <vilib>:"Read Holding Registers.vi"("error in (no error)"=w486, "quantity"=u16 5 ("number of holding registers"), "starting address"=u16 100, "MB session in"=w479) -> ("error out"=w476:errorcluster, "Registers"=w483:u16[], "MB session out"=w482:refnum<class "MB_Master.lvclass">)  [unwired: 5 in]
        n189 = case shown="无错误" w476 {
          tunnel: w483 -> [w487 _]
          frame No Error {
            n190 = global write "质控内部交互全局.vi" "总氮测量状态"(w487) -> ()
            "总氮测量状态" <- w487
          }
          frame Error {
          }
        }
        n191 = Unbundle By Name(w476) -> ("status"=w478:bool)
        n192 = Not(x=w478) -> (.not. x?=w477:bool)
        n193 = global write "质控内部交互全局.vi" "总氮通讯状态"(w477) -> ()
      }
      frame "CODMn读取" {
        n194 = property class="MB_Master"(reference=w492, "Properties:Slave ID"=u8 3 ("Slave ID")) -> (reference out=w491:refnum<class "MB_Master.lvclass">)  [unwired: 1 in, 1 out]
        n195 = call <vilib>:"Read Holding Registers.vi"("error in (no error)"=w498, "quantity"=u16 5 ("number of holding registers"), "starting address"=u16 100, "MB session in"=w491) -> ("error out"=w488:errorcluster, "Registers"=w495:u16[], "MB session out"=w494:refnum<class "MB_Master.lvclass">)  [unwired: 5 in]
        n196 = case shown="无错误" w488 {
          tunnel: w495 -> [w499 _]
          frame No Error {
            n197 = global write "质控内部交互全局.vi" "CODMn测量状态"(w499) -> ()
            "CODMn测量状态" <- w499
          }
          frame Error {
          }
        }
        n198 = Unbundle By Name(w488) -> ("status"=w490:bool)
        n199 = Not(x=w490) -> (.not. x?=w489:bool)
        n200 = global write "质控内部交互全局.vi" "CODMn通讯状态"(w489) -> ()
      }
      frame "CODCr读取" {
        n201 = property class="MB_Master"(reference=w504, "Properties:Slave ID"=u8 4 ("Slave ID")) -> (reference out=w503:refnum<class "MB_Master.lvclass">)  [unwired: 1 in, 1 out]
        n202 = call <vilib>:"Read Holding Registers.vi"("error in (no error)"=w510, "quantity"=u16 5 ("number of holding registers"), "starting address"=u16 100, "MB session in"=w503) -> ("error out"=w500:errorcluster, "Registers"=w507:u16[], "MB session out"=w506:refnum<class "MB_Master.lvclass">)  [unwired: 5 in]
        n203 = case shown="无错误" w500 {
          tunnel: w507 -> [w511 _]
          frame No Error {
            n204 = global write "质控内部交互全局.vi" "CODCr测量状态"(w511) -> ()
            "CODCr测量状态" <- w511
          }
          frame Error {
          }
        }
        n205 = Unbundle By Name(w500) -> ("status"=w502:bool)
        n206 = Not(x=w502) -> (.not. x?=w501:bool)
        n207 = global write "质控内部交互全局.vi" "CODCr通讯状态"(w501) -> ()
      }
    }
    n208 = Unbundle By Name(w420) -> ("status"=w425:bool)
    n209 = Not(x=w425) -> (.not. x?=→"通讯状态":bool)
  }
